vi "check_and_correct_input.vi"(4 "delay array":dbl[](array[numeric])) -> (1 "corrrected delay array":dbl[](array[numeric]))   [LabVIEW 2011]
doc: "Check if all the values entered by the user are correct. See the block diagram for the rules and add some if need be. \nThis vi also makes noise and shows the user what he did wrong!"
panel:
  # "check for correct data entry, \ncorrect data if necessary,\n play sound if input was wrong \nand show what was wrong"
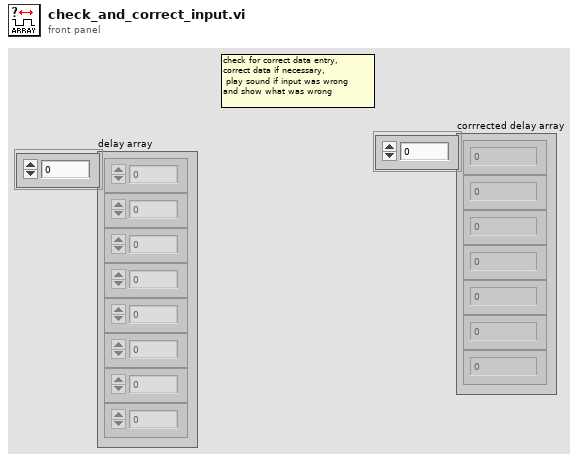
[diagram p1: front panel]
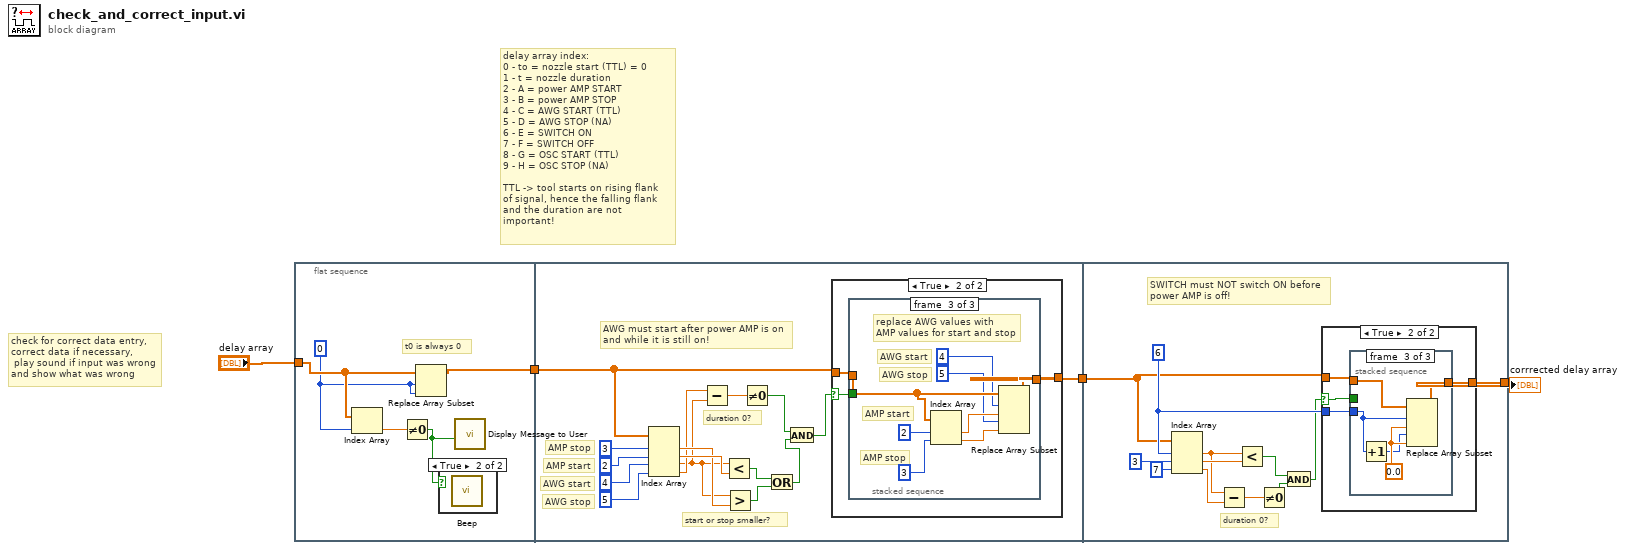
[diagram p0: block diagram]
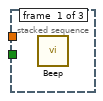
[diagram p4: hidden frame]
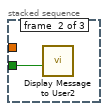
[diagram p5: hidden frame]
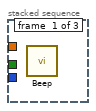
[diagram p7: hidden frame]
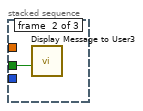
[diagram p8: hidden frame]
diagram:
  # "check for correct data entry, \ncorrect data if necessary,\n play sound if input was wrong \nand show what was wrong"
  # "delay array index:\n0 - to = nozzle start (TTL) = 0\n1 - t = nozzle duration\n2 - A = power AMP START\n3 - B = power AMP STOP\n4 - C = AWG START (TTL)\n5 - D = AWG STOP (NA)\n6 - E = SWITCH ON \n7 - F = SWITCH OFF\n8 - G = OSC START (TTL)\n9 - H = OSC STOP (NA)\n\nTTL -> tool starts on rising flank\nof signal, hence the falling flank \nand the duration are not important!"
  n1 = flat-sequence {
    tunnel: "delay array" -> [w9]
    tunnel: [w8] -> w3
    tunnel: w3 -> [w25]
    tunnel: [w23] -> w2
    tunnel: w2 -> [w48]
    tunnel: [w47] -> w1
    frame #0 {
      w6 = 0 ("index")
      # "t0 is always 0"
      n2 = Index Array(array=w9, index=w6) -> (element=w5:dbl)
      n3 = Not Equal To 0?(x=w5) -> (x != 0?=w7:bool)
      n4 = Replace Array Subset(array=w9, new element=w6, index=w6) -> (w8:dbl[])
      n5 = case shown="True" w7 {
        frame False {
        }
        frame True {
          n6 = call <vilib>:"Beep.vi"() -> ()  [unwired: 12 in]
        }
      }
      n7 = call "Display Message to User"("Enable"=w7) -> ()  [unwired: 9 in, 2 out]
    }
    frame #1 {
      # "start or stop smaller?"
      # "AWG stop"
      # "AWG start"
      # "AMP stop"
      # "AMP start"
      # "duration 0?"
      # "AWG must start after power AMP is on \nand while it is still on!"
      n8 = Index Array(array=w25, index #1=3 ("index"), index #2=2 ("index"), index #3=4 ("index"), index #4=5 ("index")) -> (element #1=w17:dbl, element #2=w18:dbl, element #3=w10:dbl, element #4=w11:dbl)
      n9 = Subtract(x=w11, y=w10) -> (x-y=w21:dbl)
      n10 = Less?(x=w10, y=w18) -> (x < y?=w16:bool)
      n11 = Greater?(x=w10, y=w17) -> (0:w15:bool)
      n12 = Not Equal To 0?(x=w21) -> (x != 0?=w14:bool)
      n13 = Or(x=w16, y=w15) -> (x .or. y?=w13:bool)
      n14 = And(x=w14, y=w13) -> (x .and. y?=w12:bool)
      n15 = case shown="True" w12 {
        selector: w12 -> [_ w29]
        tunnel: [w26 w28] -> w23
        tunnel: w25 -> [w26 w27]
        frame False {
        }
        frame True {
          n16 = stacked-sequence {
            tunnel: w29 -> [_ w30 _]
            tunnel: [_ _ w38] -> w28
            tunnel: w27 -> [_ _ w35]
            frame #0 {
              n17 = call <vilib>:"Beep.vi"() -> ()  [unwired: 12 in]
            }
            frame #1 {
              n18 = call "Display Message to User2"("Enable"=w30) -> ()  [unwired: 9 in, 2 out]
            }
            frame #2 {
              # "replace AWG values with \nAMP values for start and stop"
              # "AWG stop"
              # "AWG start"
              # "AMP start"
              # "AMP stop"
              n19 = Index Array(array=w35, index #1=2 ("index"), index #2=3 ("index")) -> (element #1=w33:dbl, element #2=w32:dbl)
              n20 = Replace Array Subset(array=w35, new element #1=w33, index #1=4 ("index"), new element #2=w32, index #2=5 ("index")) -> (w38:dbl[])
            }
          }
        }
      }
    }
    frame #2 {
      w49 = 6 ("index")
      # "duration 0?"
      # "SWITCH must NOT switch ON before \npower AMP is off!"
      n21 = Index Array(array=w48, index #1=w49, index #2=3 ("index"), index #3=7 ("index")) -> (element #1=w44:dbl, element #2=w46:dbl, element #3=w43:dbl)
      n22 = Subtract(x=w44, y=w43) -> (x-y=w42:dbl)
      n23 = Less?(x=w44, y=w46) -> (x < y?=w40:bool)
      n24 = Not Equal To 0?(x=w42) -> (x != 0?=w41:bool)
      n25 = And(x=w40, y=w41) -> (x .and. y?=w39:bool)
      n26 = case shown="True" w39 {
        selector: w39 -> [_ w55]
        tunnel: [w51 w54] -> w47
        tunnel: w48 -> [w51 w53]
        tunnel: w49 -> [_ w52]
        frame False {
        }
        frame True {
          n27 = stacked-sequence {
            tunnel: w55 -> [_ w56 _]
            tunnel: [_ _ w61] -> w54
            tunnel: w53 -> [_ _ w59]
            tunnel: w52 -> [_ _ w58]
            frame #0 {
              n28 = call <vilib>:"Beep.vi"() -> ()  [unwired: 12 in]
            }
            frame #1 {
              n29 = call "Display Message to User3"("Enable"=w56) -> ()  [unwired: 9 in, 2 out]
            }
            frame #2 {
              w60 = 0.0 ("new element/subarray")
              n30 = Increment(x=w58) -> (x+1=w57:i32)
              n31 = Replace Array Subset(array=w59, new element #1=w60, index #1=w58, new element #2=w60, index #2=w57) -> (w61:dbl[])
            }
          }
        }
      }
    }
  }
  "corrrected delay array" <- w1
